vi "Regler Verwaltung.vi"() -> (0 "error out":errorcluster caption="Fehler (Ausgang)")   [LabVIEW 2020, in "Regler.lvlib"]
uses:
  Regler.lvlib
  FGV Daten Regler Aktionen.ctl
  Allgemein/FGV Zustaende Aktionen.ctl
  Funktionstasten/Zustaende.ctl
  Verwaltung/FGV IN Aktionen.ctl
  Konfig-Dateien/FGV Betriebsdaten Aktionen.ctl
  Verwaltung/Verwaltung - cRIO.lvlib
  Konfig-Dateien/Konfig-Dateien.lvlib
  Allgemein/Allgemein.lvlib
  Funktionstasten/Funktionstasten.lvlib
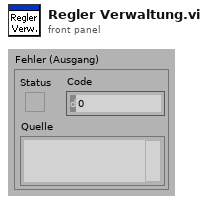
[diagram p1: front panel]
types:
  T1 = typedef "Regler.lvlib/FGV Daten Regler Aktionen.ctl" = enum16{"lesen", "Out%", "Heizung EIN"}
  T2 = typedef "Konfig-Dateien.lvlib/FGV Betriebsdaten Aktionen.ctl" = enum16{"lesen", "Anlagengrenzw.", "PID Param.", "Sonstige", "Sensor Para."}
  T3 = typedef "Verwaltung - cRIO.lvlib/FGV IN Aktionen.ctl" = enum16{"lesen", "DI", "AI", "Fühler Br.", "TC", "Fühler Br. TC"}
  T4 = typedef "Funktionstasten.lvlib/Zustaende.ctl" = enum16{"Standby", "Pause", "Eco", "Messen", "Kalibrieren", "Spülen Filter", "Spülen Leitung", "Umgebungsluft", "0-Gas", "Cal-Gas", "CG zu PNS", "-------------", "Init 1", "Init 2", "Init 3", "Init 4", "Messen vorbereiten", "Messen durchführen", "Exit"}
  T5 = typedef "Allgemein.lvlib/FGV Zustaende Aktionen.ctl" = enum16{"lesen", "Zustand PC", "Zustand cRIO", "Bildnummer", "Samplepoint", "Sysloglevel"}
  T6 = typedef "Erweiterte Konfig.lvlib/PID-Parameter Anzeige.ctl" = cluster{"Heizung\nFilterblock":T7, "Heizung\nPumpe":T7, "Heizung\nHeizleitungen":T7, "Heizleitung\nExtern":T7, "Heizung\nFB-Druckregler":T7}
  T7 = typedef "Erweiterte Konfig.lvlib/PID-Parameter.ctl" = cluster{"P-Anteil":T8, "I-Anteil":T8, "D-Anteil":T8, "Regelzonengr.":T8, "max. OUT":T8}
  T8 = typedef "Zahlen-Eingabefeld.ctl" = sgl
  T9 = typedef "Anlagengrenzwerte.lvlib/Anlagen-Grenzwerte Anzeige.ctl" = cluster{"Eingangsdruck FT-IR:":T10, "Durchfluss FT-IR:":T10, "Durchfluss CalGas:":T10, "Druck Ausgang:":T10, "Druck Kalter Block:":T10, "Heizleitungen intern:":T10, "Heizleitung zu FT-IR:":T10, "Heizung Filterblock:":T10, "Heizung Pumpe:":T10, "Heizleitung Extern SP1:":T10, "Heizleitung Extern SP2:":T10, "FT-IR Heizung Messzelle:":T10, "Schaltschranktemperatur:":T10, "Gaskühler:":T10}
  T10 = typedef "Anlagengrenzwerte.lvlib/Anlagen-Parameter Anzeige.ctl" = cluster{"Sollwert":sgl, "Warn-Min":sgl, "Warn-Max":sgl, "Abschalt-Min":sgl, "Abschalt-Max":sgl, "Regler":u16}
  T11 = typedef "Verwaltung - cRIO.lvlib/TC Eingaenge.ctl" = cluster{"TC0: Reserve":sgl, "TC1: HL zu FT-IR":sgl, "TC2: HL Extern SP1":sgl, "TC3: HL Extern SP2":sgl, "TC4: Reserve":sgl, "TC5: Reserve":sgl, "TC6: Reserve":sgl, "TC7: Reserve":sgl, "TC8: FT-IR":sgl, "TC9: Reserve":sgl, "TC10: Schaltschrank":sgl, "TC11: Umgebung":sgl}
  T12 = typedef "Verwaltung - cRIO.lvlib/Fuehler Bruch TC.ctl" = cluster{"TC0: Reserve":bool, "TC1: HL zu FT-IR":bool, "TC2: HL Extern SP1":bool, "TC3: HL Extern SP2":bool, "TC4: Reserve":bool, "TC5: Reserve":bool, "TC6: Reserve":bool, "TC7: Reserve":bool, "TC8: FT-IR":bool, "TC9: Reserve":bool, "TC10: Schaltschrank":bool, "TC11: Umgebung":bool}
  T13 = cluster{"Output% 1":i16, "Output% 2":i16, "Output% 3":i16, "Output% 4":i16, "Output% 5":i16, "Output% 6":i16, "Output% 7":i16, "Output% 8":i16, "Output% 9":i16, "Output% 10":i16, "Output% 11":i16, "Output% 12":i16, "Output% 13":i16, "Output% 14":i16, "Output% 15":i16, "Output% 16":i16, "Output% 17":i16, "Output% 18":i16}
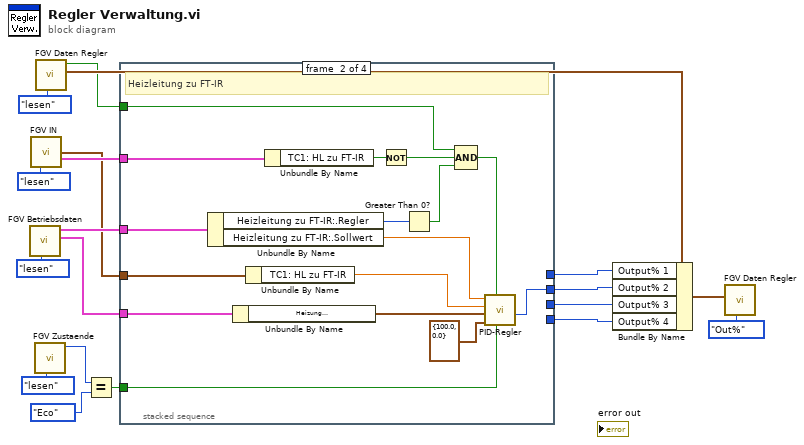
[diagram p0: block diagram]
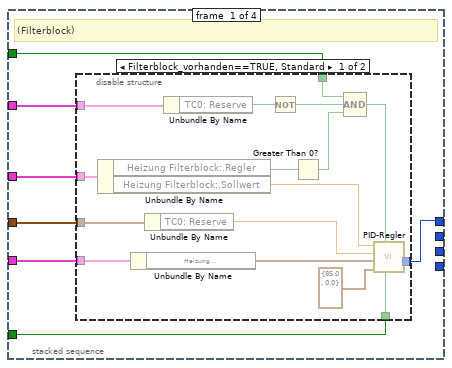
[diagram p2: hidden frame]
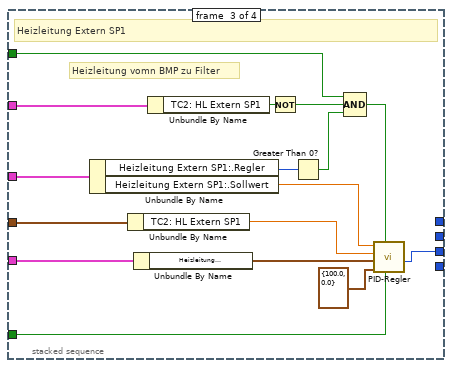
[diagram p4: hidden frame]
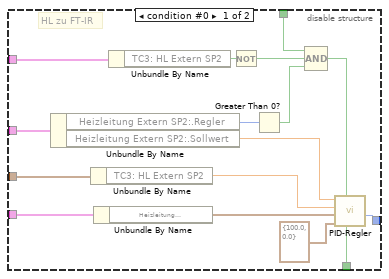
[diagram p6: hidden frame]
diagram:
  n1 = call "FGV Betriebsdaten.vi"("Aktionen"=FGV_Betriebsdaten_Aktionen."lesen") -> ("PID-Parameter"=w5:T6, "Anlagen-Grenzwerte"=w6:T9)  [unwired: 7 in, 2 out]
  n2 = call "FGV IN.vi"("Aktion"=FGV_IN_Aktionen."lesen") -> ("TC Eingänge"=w1:T11, "Fühler Bruch TC"=w2:T12)  [unwired: 10 in, 3 out]
  n3 = call "FGV Zustaende.vi"("Aktionen"=FGV_Zustaende_Aktionen."lesen") -> ("Zustand PC"=w10:T4)  [unwired: 6 in, 4 out]
  n4 = call "FGV Daten Regler.vi"("Aktionen"=FGV_Daten_Regler_Aktionen."lesen") -> ("PID - OUT%"=w13:T13, "Heizung EIN"=w12:bool)  [unwired: 9 in]
  n5 = Equal?(x=w10, y=Zustaende."Eco") -> (x = y?=w15:bool)
  n6 = stacked-sequence {
    tunnel: w6 -> [w26 w58 w74 w81]
    tunnel: w1 -> [w25 w57 w73 w80]
    tunnel: [w24 _ _ _] -> w19
    tunnel: w5 -> [w23 w44 w70 w79]
    tunnel: [_ w45 _ _] -> w18
    tunnel: [_ _ w59 _] -> w17
    tunnel: [_ _ _ w75] -> w16
    tunnel: w2 -> [w22 w54 w68 w78]
    tunnel: w12 -> [w21 w51 w65 w77]
    tunnel: w15 -> [w20 w46 w60 w76]
    frame #0 {
      # "(Filterblock)"
      n7 = disable-structure shown="Filterblock_vorhanden==TRUE, Standard" {
        disable-tunnel: w26 -> [w42 _]
        disable-tunnel: w25 -> [w41 _]
        disable-tunnel: [w38 _] -> w24
        disable-tunnel: w23 -> [w37 _]
        disable-tunnel: w22 -> [w35 _]
        disable-tunnel: w21 -> [w32 _]
        disable-tunnel: w20 -> [w27 _]
        frame condition #0 {
          n8 = Unbundle By Name(w42) -> ("Heizung Filterblock:.Regler"=w30:u16, "Heizung Filterblock:.Sollwert"=w40:sgl)
          n9 = Unbundle By Name(w37) -> ("Heizung\nFilterblock"=w36:T7)
          n10 = Unbundle By Name(w41) -> ("TC0: Reserve"=w39:sgl)
          n11 = Unbundle By Name(w35) -> ("TC0: Reserve"=w34:bool)
          n12 = Not(x=w34) -> (.not. x?=w31:bool)
          n13 = Greater Than 0?(x=w30) -> (x > 0?=w29:bool)
          n14 = Compound Arithmetic op=AND(w32, w31, w29) -> (w28:bool)
          n15 = call "PID-Regler.vi"("ECO Mode"=w27, "Regler EIN"=w28, "Output Range"=cluster{"Output High":sgl, "Output Low":sgl} {"Output High"=85.0, "Output Low"=0.0}, "PID-Parameter"=w36, "Istwert"=w39, "Sollwert"=w40) -> ("Output"=w38:i16)  [unwired: 5 out]
        }
        frame condition #1 (active) {
        }
      }
    }
    frame #1 {
      # "Heizleitung zu FT-IR"
      n16 = Unbundle By Name(w58) -> ("Heizleitung zu FT-IR:.Regler"=w49:u16, "Heizleitung zu FT-IR:.Sollwert"=w56:sgl)
      n17 = Unbundle By Name(w44) -> ("Heizung\nHeizleitungen"=w43:T7)
      n18 = Unbundle By Name(w57) -> ("TC1: HL zu FT-IR"=w55:sgl)
      n19 = Unbundle By Name(w54) -> ("TC1: HL zu FT-IR"=w53:bool)
      n20 = Not(x=w53) -> (.not. x?=w50:bool)
      n21 = Greater Than 0?(x=w49) -> (x > 0?=w48:bool)
      n22 = Compound Arithmetic op=AND(w51, w50, w48) -> (w47:bool)
      n23 = call "PID-Regler.vi"("ECO Mode"=w46, "Regler EIN"=w47, "Output Range"=cluster{"Output High":sgl, "Output Low":sgl} {"Output High"=100.0, "Output Low"=0.0}, "PID-Parameter"=w43, "Istwert"=w55, "Sollwert"=w56) -> ("Output"=w45:i16)  [unwired: 5 out]
    }
    frame #2 {
      # "Heizleitung vomn BMP zu Filter"
      # "Heizleitung Extern SP1"
      n24 = Unbundle By Name(w74) -> ("Heizleitung Extern SP1:.Regler"=w63:u16, "Heizleitung Extern SP1:.Sollwert"=w72:sgl)
      n25 = Unbundle By Name(w73) -> ("TC2: HL Extern SP1"=w71:sgl)
      n26 = Unbundle By Name(w70) -> ("Heizleitung\nExtern"=w69:T7)
      n27 = Unbundle By Name(w68) -> ("TC2: HL Extern SP1"=w67:bool)
      n28 = Not(x=w67) -> (.not. x?=w64:bool)
      n29 = Greater Than 0?(x=w63) -> (x > 0?=w62:bool)
      n30 = Compound Arithmetic op=AND(w65, w64, w62) -> (w61:bool)
      n31 = call "PID-Regler.vi"("ECO Mode"=w60, "Regler EIN"=w61, "Output Range"=cluster{"Output High":sgl, "Output Low":sgl} {"Output High"=100.0, "Output Low"=0.0}, "PID-Parameter"=w69, "Istwert"=w71, "Sollwert"=w72) -> ("Output"=w59:i16)  [unwired: 5 out]
    }
    frame #3 {
      # "Heizleitung Extern SP2"
      n32 = disable-structure shown="Heizleitung_SP2==FALSE" {
        disable-tunnel: w81 -> [w97 _]
        disable-tunnel: w80 -> [w96 _]
        disable-tunnel: w79 -> [w93 _]
        disable-tunnel: w78 -> [w91 _]
        disable-tunnel: w77 -> [w88 _]
        disable-tunnel: w76 -> [w83 _]
        disable-tunnel: [w82 _] -> w75
        frame condition #0 {
          # "HL zu FT-IR"
          n33 = Unbundle By Name(w97) -> ("Heizleitung Extern SP2:.Regler"=w86:u16, "Heizleitung Extern SP2:.Sollwert"=w95:sgl)
          n34 = Unbundle By Name(w96) -> ("TC3: HL Extern SP2"=w94:sgl)
          n35 = Unbundle By Name(w93) -> ("Heizleitung\nExtern"=w92:T7)
          n36 = Unbundle By Name(w91) -> ("TC3: HL Extern SP2"=w90:bool)
          n37 = Not(x=w90) -> (.not. x?=w87:bool)
          n38 = Greater Than 0?(x=w86) -> (x > 0?=w85:bool)
          n39 = Compound Arithmetic op=AND(w88, w87, w85) -> (w84:bool)
          n40 = call "PID-Regler.vi"("ECO Mode"=w83, "Regler EIN"=w84, "Output Range"=cluster{"Output High":sgl, "Output Low":sgl} {"Output High"=100.0, "Output Low"=0.0}, "PID-Parameter"=w92, "Istwert"=w94, "Sollwert"=w95) -> ("Output"=w82:i16)  [unwired: 5 out]
        }
        frame condition #1 (active) {
        }
      }
    }
  }
  n41 = Bundle By Name(cluster=w13, "Output% 1"=w19, "Output% 2"=w18, "Output% 3"=w17, "Output% 4"=w16) -> (w3:T13)
  n42 = call "FGV Daten Regler.vi"("Aktionen"=FGV_Daten_Regler_Aktionen."Out%", "PID - OUT%"=w3) -> ()  [unwired: 8 in, 2 out]
